vi "PatternDialog.vi"(8 "Error In":errorcluster {"code" format="%.0x"}, 10 "Default Pattern Folder":path=path "" caption="start path", 11 "Pattern In":T10) -> (0 "Error Out":errorcluster {"code" format="%.0x"}, 2 "Cancelled?":bool, 3 "Pattern Out":T10)   [LabVIEW 2012, in "Virtual-PGA.lvlib"]
doc: "This VI provides a dialog for creating, loading, and saving patterns from within other applications."
uses:
  Virtual-PGA.lvlib
  Controls/Pattern.ctl
  Controls/Input.ctl
  Controls/64PinPGAPattern.ctl
  Controls/64PinPGAPads1-16.ctl
  Controls/64PinPGAPad1-16.ctl
  Controls/64PinPGAPads17-32.ctl
  Controls/64PinPGAPad17-32.ctl
  Controls/64PinPGAPads33-48.ctl
  Controls/64PinPGAPad33-48.ctl
  Controls/64PinPGAPads49-64.ctl
  Controls/64PinPGAPad49-64.ctl
panel:
  in  "64-Pin PGA":T1
  in  "RESET":bool
  in  "SAVE":bool
  in  "CANCEL":bool
  in  "DONE":bool
  in  "LOAD":bool
  # "Name:"
  # "Inputs:"
  # "Description:"
  # "Y4:"
  # "Y3:"
  # "Y2:"
  # "Y1:"
  # "49"
  # "50"
  # "51"
  # "52"
  # "53"
  # "54"
  # "55"
  # "56"
  # "57"
  # "58"
  # "59"
  # "60"
  # "61"
  # "62"
  # "63"
  # "64"
  # "1"
  # "2"
  # "3"
  # "4"
  # "5"
  # "6"
  # "7"
  # "8"
  # "9"
  # "10"
  # "11"
  # "12"
  # "13"
  # "14"
  # "15"
  # "16"
  # "32"
  # "31"
  # "30"
  # "29"
  # "28"
  # "27"
  # "26"
  # "25"
  # "24"
  # "23"
  # "22"
  # "21"
  # "20"
  # "19"
  # "18"
  # "17"
  # "48"
  # "47"
  # "46"
  # "45"
  # "44"
  # "43"
  # "42"
  # "41"
  # "40"
  # "39"
  # "38"
  # "37"
  # "36"
  # "35"
  # "34"
  # "33"
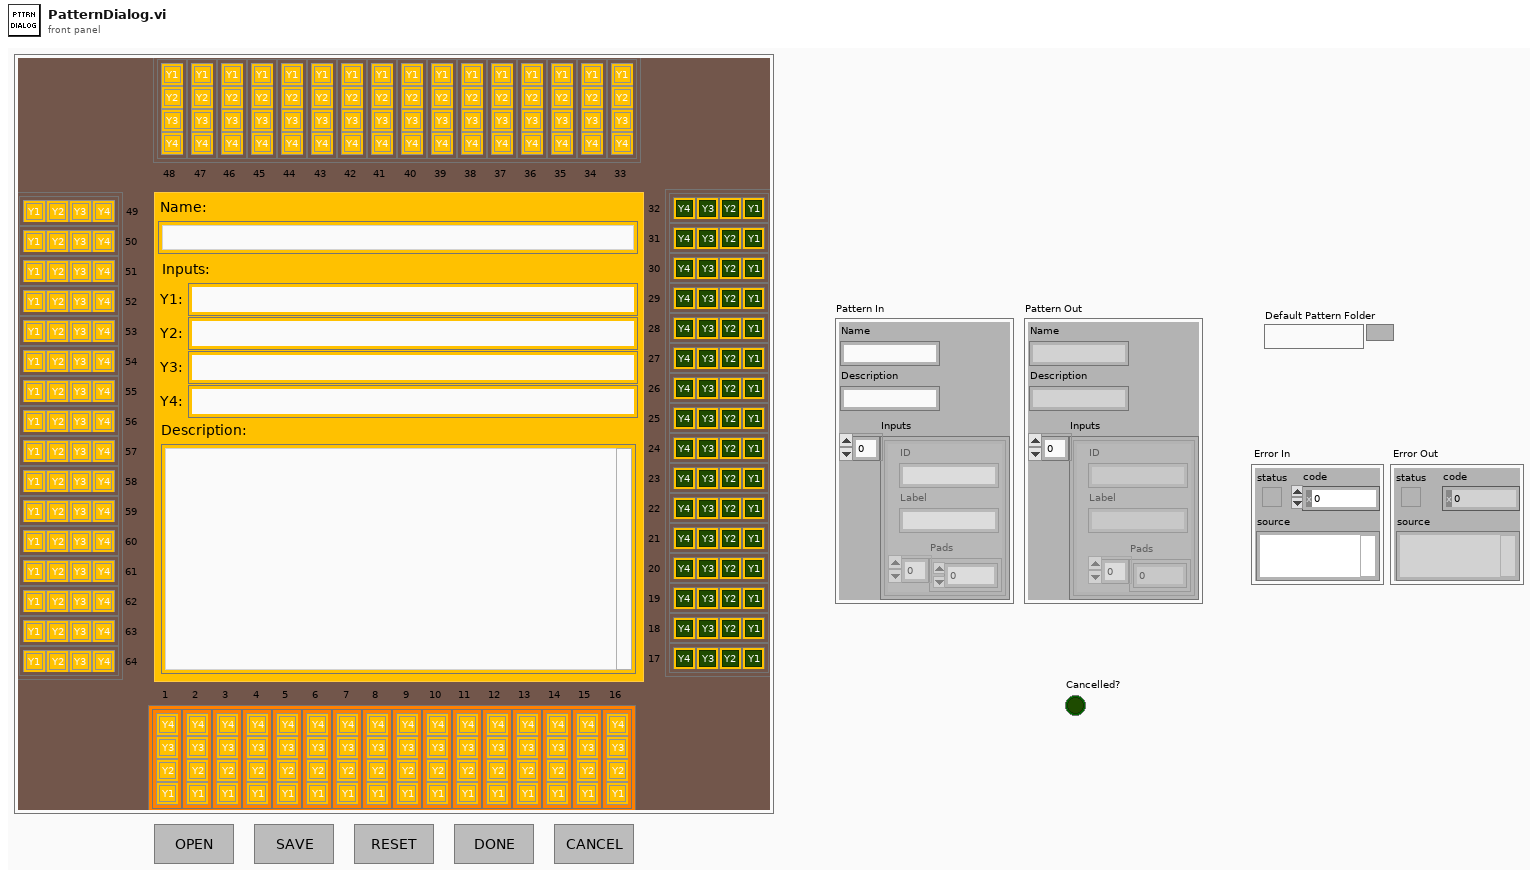
[diagram p1: front panel]
types:
  T1 = typedef "Virtual-PGA.lvlib/64PinPGAPattern.ctl" = cluster{"Name":string, "Description":string, "Y1 Label":string, "Y2 Label":string, "Y3 Label":string, "Y4 Label":string, "Pads 1-16":T2, "Pads 17-32":T4, "Pads 33-48":T6, "Pads 49-64":T8}
  T2 = typedef "Virtual-PGA.lvlib/64PinPGAPads1-16.ctl" = T3[]
  T3 = typedef "Virtual-PGA.lvlib/64PinPGAPad1-16.ctl" = cluster{"Y1":bool, "Y2":bool, "Y3":bool, "Y4":bool}
  T4 = typedef "Virtual-PGA.lvlib/64PinPGAPads17-32.ctl" = T5[]
  T5 = typedef "Virtual-PGA.lvlib/64PinPGAPad17-32.ctl" = cluster{"Y1":bool, "Y2":bool, "Y3":bool, "Y4":bool}
  T6 = typedef "Virtual-PGA.lvlib/64PinPGAPads33-48.ctl" = T7[]
  T7 = typedef "Virtual-PGA.lvlib/64PinPGAPad33-48.ctl" = cluster{"Y1":bool, "Y2":bool, "Y3":bool, "Y4":bool}
  T8 = typedef "Virtual-PGA.lvlib/64PinPGAPads49-64.ctl" = T9[]
  T9 = typedef "Virtual-PGA.lvlib/64PinPGAPad49-64.ctl" = cluster{"Y1":bool, "Y2":bool, "Y3":bool, "Y4":bool}
  T10 = typedef "Virtual-PGA.lvlib/Pattern.ctl" = cluster{"Name":string, "Description":string, "Inputs":T11[]}
  T11 = typedef "Virtual-PGA.lvlib/Input.ctl" = cluster{"ID":string, "Label":string, "Pads":u32[]}
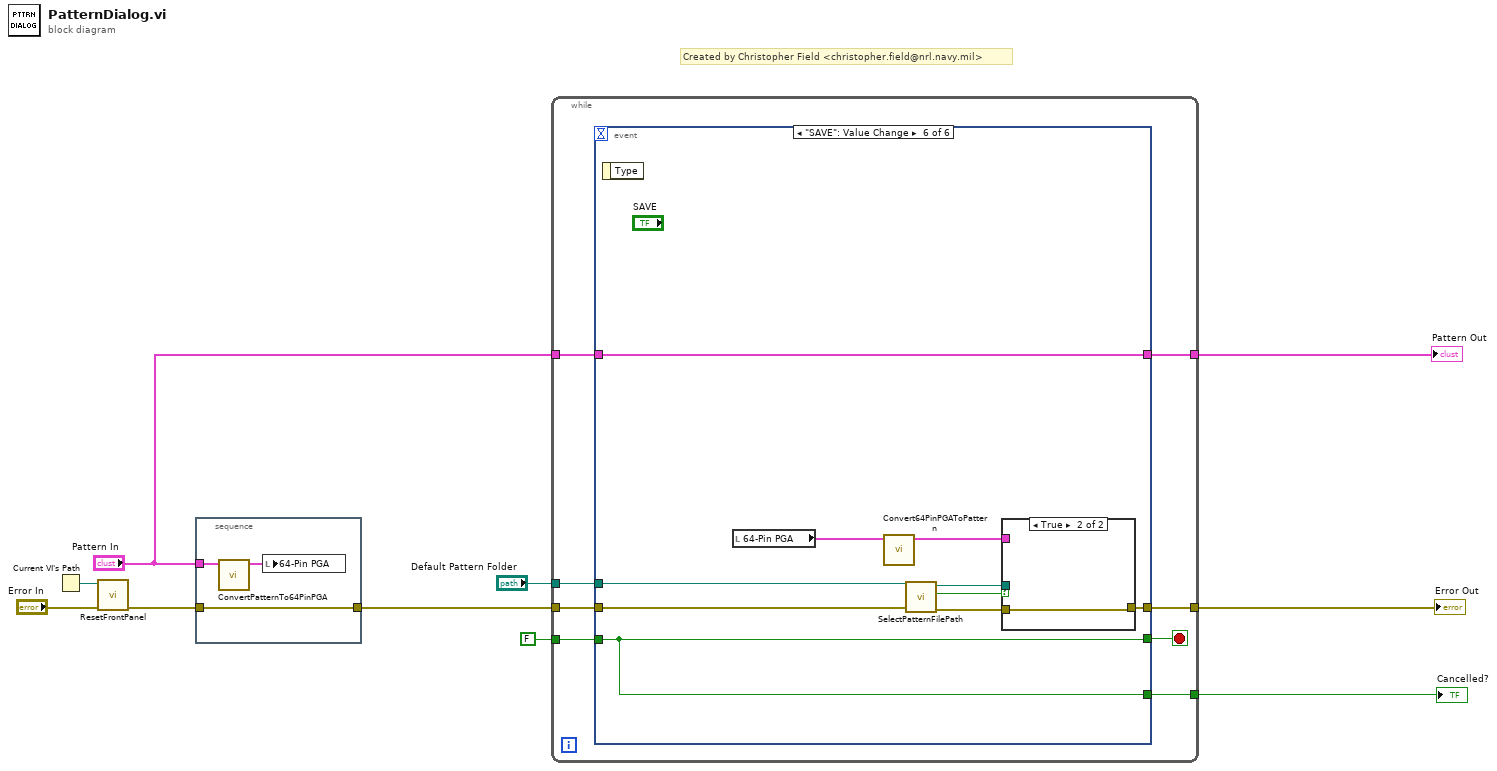
[diagram p0: block diagram]
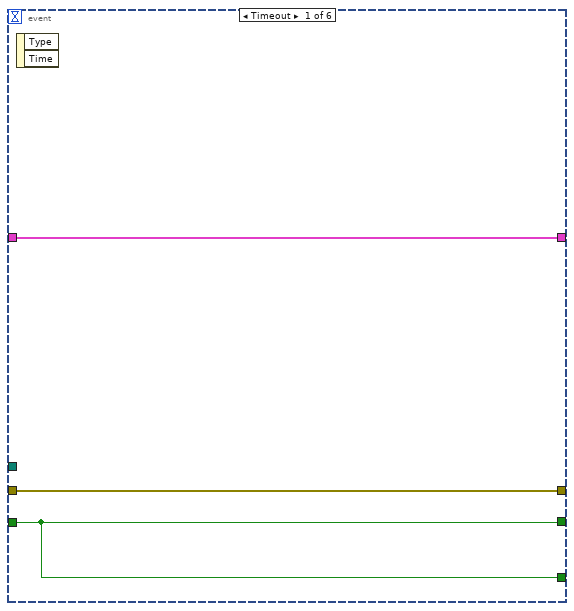
[diagram p2: hidden frame]
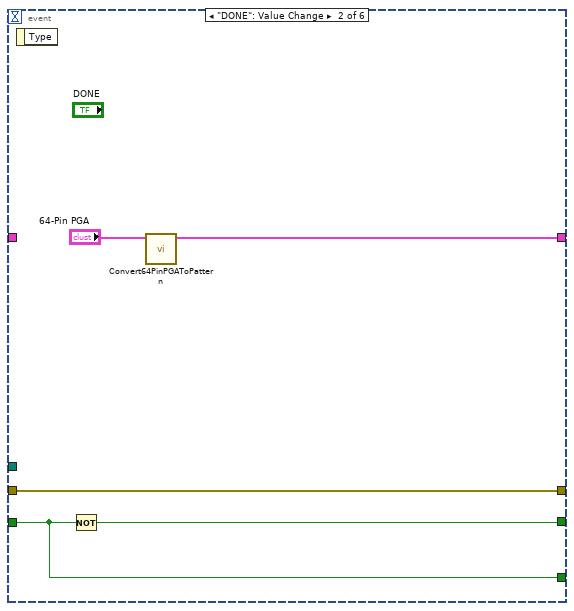
[diagram p3: hidden frame]
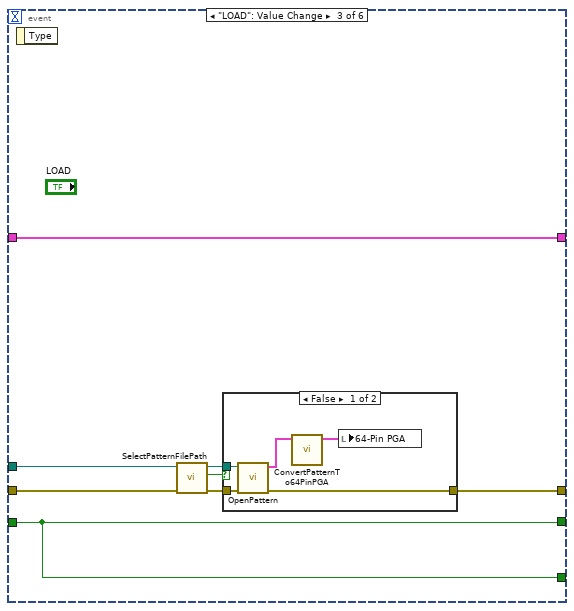
[diagram p4: hidden frame]
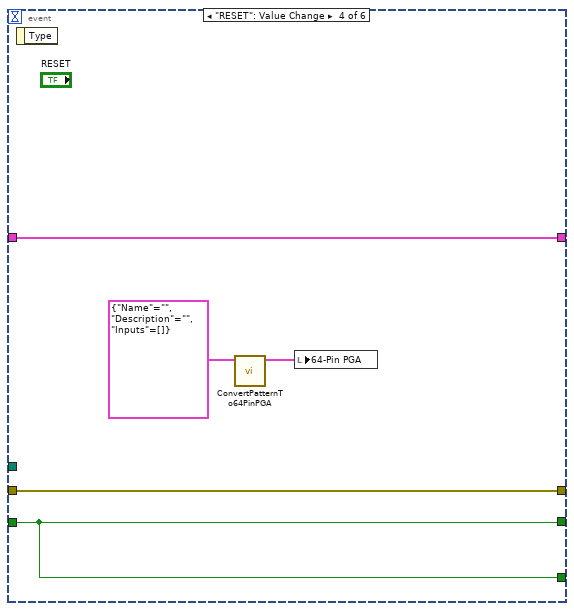
[diagram p6: hidden frame]
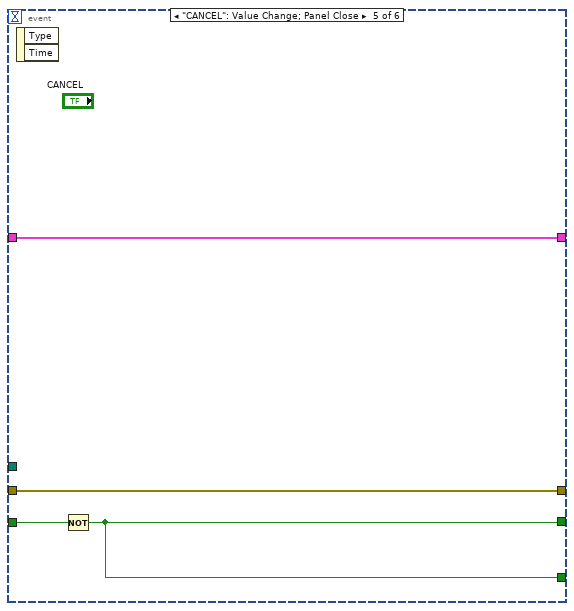
[diagram p7: hidden frame]
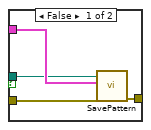
[diagram p8: hidden frame]
diagram:
  # "Created by Christopher Field <christopher.field@nrl.navy.mil>"
  n1 = Current VI's Path() -> (path=w6:path)
  n2 = call "ResetFrontPanel.vi"("Error In"="Error In", "VI Path"=w6) -> ("Error Out"=w5:errorcluster)  [unwired: 9 in]
  n3 = stacked-sequence {
    tunnel: w5 -> [w13]
    tunnel: [w13] -> w4
    tunnel: "Pattern In" -> [w11]
    frame #0 {
      n4 = call "ConvertPatternTo64PinPGA.vi"("Pattern"=w11) -> ("64-Pin PGA"=w12:T1)  [unwired: 10 in]
      n5 = local write "64-Pin PGA"(w12) -> ()
    }
  }
  n6 = while {
    tunnel: FALSE -> [w20]
    tunnel: w4 -> [w19]
    tunnel: [w18] -> w9
    tunnel: [w17] -> w8
    tunnel: [w16] -> w3
    tunnel: "Pattern In" -> [w15]
    tunnel: "Default Pattern Folder" -> [w14]
    stop <- w21 stop-if-true
    n7 = event shown="[5] \"SAVE\": Value Change" {
      selector: _ -> [_ _ _ _ _ _]
      dyn-events: _ -> [_ _ _ _ _ _]
      timeout: _ -> [_ _ _ _ _ _]
      tunnel: [w23 w29 w37 w47 w50 w61] -> w21
      tunnel: w20 -> [w23 w27 w37 w47 w51 w61]
      tunnel: w19 -> [w24 w28 w30 w48 w52 w54]
      tunnel: [w24 w28 w36 w48 w52 w62] -> w18
      tunnel: [w23 w27 w37 w47 w50 w61] -> w17
      tunnel: [w22 w25 w35 w44 w49 w58] -> w16
      tunnel: w15 -> [w22 _ w35 w44 w49 w58]
      tunnel: w14 -> [_ _ w31 _ _ w53]
      event Timeout {
        n8 = event-data() -> ()  [unwired: 1 in, 2 out]
      }
      event "DONE": Value Change {
        n9 = event-data() -> ()  [unwired: 1 in, 1 out]
        n10 = Not(x=w27) -> (.not. x?=w29:bool)
        n11 = call "Convert64PinPGAToPattern.vi"("64-Pin PGA"="64-Pin PGA") -> ("Pattern"=w25:T10)  [unwired: 10 in]
      }
      event "LOAD": Value Change {
        n12 = event-data() -> ()  [unwired: 1 in, 1 out]
        n13 = call "SelectPatternFilePath.vi"("Error In"=w30, "Start Path"=w31) -> ("Error Out"=w32:errorcluster, "Cancelled?"=w33:bool, "Pattern Path"=w34:path)  [unwired: 7 in]
        n14 = case shown="False" w33 {
          tunnel: [w42 w43] -> w36
          tunnel: w32 -> [w41 w43]
          tunnel: w34 -> [w40 _]
          frame False {
            n15 = call "OpenPattern.vi"("Error In"=w41, "Patten File Path"=w40) -> ("Error Out"=w42:errorcluster, "Pattern"=w39:T10)  [unwired: 8 in]
            n16 = call "ConvertPatternTo64PinPGA.vi"("Pattern"=w39) -> ("64-Pin PGA"=w38:T1)  [unwired: 10 in]
            n17 = local write "64-Pin PGA"(w38) -> ()
          }
          frame True {
          }
        }
      }
      event "RESET": Value Change {
        n18 = event-data() -> ()  [unwired: 1 in, 1 out]
        n19 = call "ConvertPatternTo64PinPGA.vi"("Pattern"=T10 {"Name"="", "Description"="", "Inputs"=[]} ("Pattern In")) -> ("64-Pin PGA"=w45:T1)  [unwired: 10 in]
        n20 = local write "64-Pin PGA"(w45) -> ()
      }
      event "CANCEL": Value Change; Panel Close {
        n21 = event-data() -> ()  [unwired: 1 in, 2 out]
        n22 = Not(x=w51) -> (.not. x?=w50:bool)
      }
      event "SAVE": Value Change {
        n23 = event-data() -> ()  [unwired: 1 in, 1 out]
        n24 = local read "64-Pin PGA"() -> (w59:T1)
        n25 = call "Convert64PinPGAToPattern.vi"("64-Pin PGA"=w59) -> ("Pattern"=w60:T10)  [unwired: 10 in]
        n26 = call "SelectPatternFilePath.vi"("Error In"=w54, "Start Path"=w53) -> ("Error Out"=w55:errorcluster, "Cancelled?"=w57:bool, "Pattern Path"=w56:path)  [unwired: 7 in]
        n27 = case shown="True" w57 {
          tunnel: [w66 w67] -> w62
          tunnel: w60 -> [w65 _]
          tunnel: w56 -> [w64 _]
          tunnel: w55 -> [w63 w67]
          frame False {
            n28 = call "SavePattern.vi"("Error In"=w63, "Pattern"=w65, "Pattern Save Path"=w64) -> ("Error Out"=w66:errorcluster)  [unwired: 7 in, 1 out]
          }
          frame True {
          }
        }
      }
    }
  }
  "Error Out" <- w9
  "Pattern Out" <- w3
  "Cancelled?" <- w8
